vi "Thread Error Handler.vi"(8 "error in (no error)":errorcluster, 11 "Thread in":refnum<class "Thread.lvclass">) -> (0 "error out":errorcluster, 3 "Thread out":refnum<class "Thread.lvclass">)   [LabVIEW 2016, in "Architecture.lvlib" / "Thread.lvclass"]
uses:
  Thread.lvclass
  Error Handler/EH Action.ctl
  Error Handler/Error Handler.lvclass
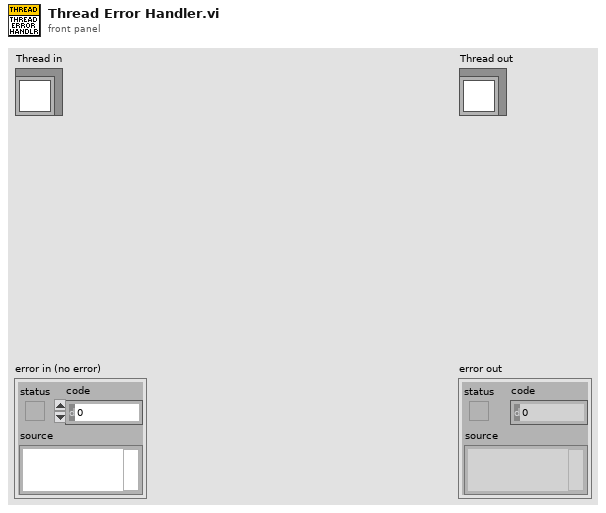
[diagram p1: front panel]
types:
  T1 = typedef "Architecture.lvlib/Error Handler.lvclass/EH Action.ctl" = enum16{"Define Threads", "Close", "System Error", "Wash Cycle Error", "Minor Error", "Initialize"}
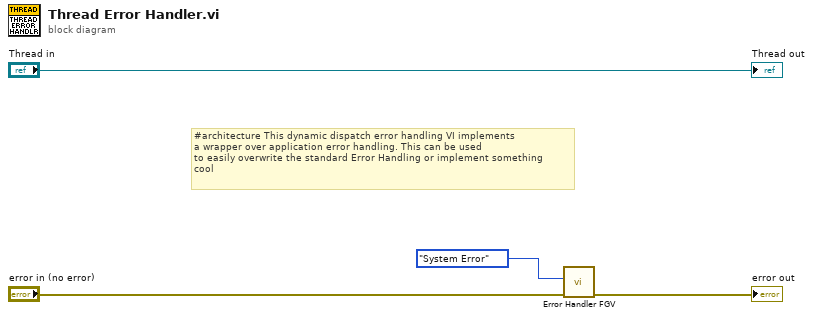
[diagram p0: block diagram]
diagram:
  # "#architecture This dynamic dispatch error handling VI implements\na wrapper over application error handling. This can be used\nto easily overwrite the standard Error Handling or implement something\ncool"
  n1 = call "Error Handler FGV.vi"("error in (no error)"="error in (no error)", "Action"=EH_Action."System Error") -> ("error out"=→"error out":errorcluster)  [unwired: 9 in]
  "Thread out" <- "Thread in"
